vi "p1.vi"() -> ()   [LabVIEW 2021, in "d14.lvlib"]
uses:
  d14.lvlib
  AOC/AOC.lvlib
panel:
  out "XY Graph":cluster{"Left out":u32[], "Top out":u32[]}[](graph)
  out "Answer":i32
  in  "Example":string="498,4 -> 498,6 -> 496,6\n503,4 -> 502,4 -> 502,9 -> 494,9"
  in  "Example":bool
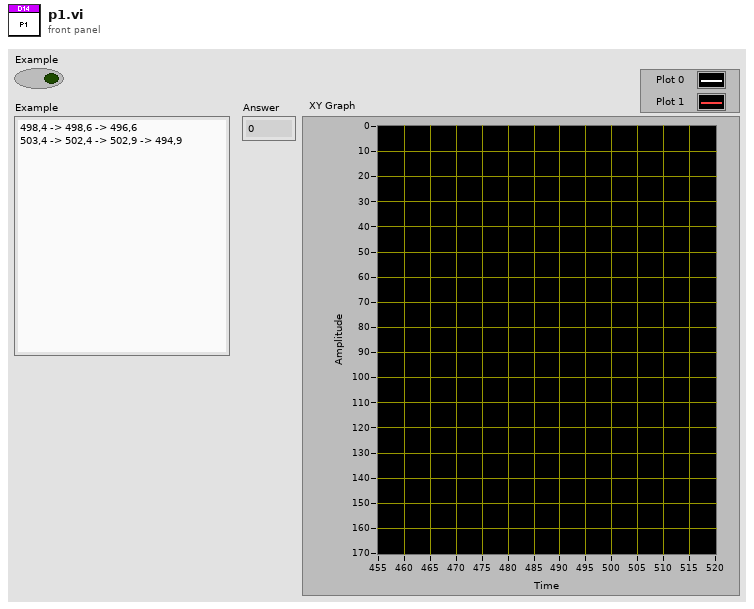
[diagram p1: front panel]
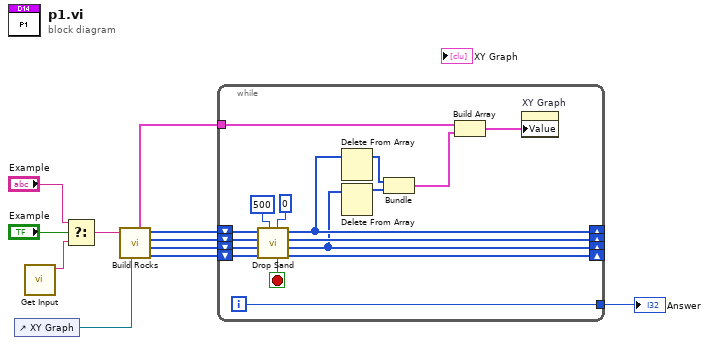
[diagram p0: block diagram]
diagram:
  n1 = control-ref of="XY Graph"() -> (w1:refnum<vi>)
  n2 = call "Get Input.vi"() -> ("Input"=w11:string)  [unwired: 11 in]
  n3 = Select(t="Example", s="Example", f=w11) -> (s? t:f=w10:string)
  n4 = call "Build Rocks.vi"("reference"=w1, "Input"=w10) -> ("Bottom"=w3:i32[], "Top"=w5:i32[], "Right"=w4:i32[], "Left"=w6:i32[], "Rocks"=w2:cluster{u32[], u32[]})  [unwired: 4 in, 1 out]
  n5 = while {
    tunnel: [w23] -> w7
    shift-right: [w18] -> _
    shift-left: w6 -> [w27]
    shift-right: [w20] -> _
    shift-left: w4 -> [w26]
    shift-right: [w17] -> _
    shift-left: w5 -> [w28]
    shift-right: [w19] -> _
    shift-left: w3 -> [w25]
    tunnel: w2 -> [w14]
    i -> [w23]
    stop <- w24 stop-if-true
    n6 = call "Drop Sand.vi"("Y in"=0, "X in"=500, "Bottom in"=w25, "Top in"=w28, "Right in"=w26, "Left in"=w27) -> ("Bottom out"=w19:i32[], "Top out"=w17:i32[], "Right out"=w20:i32[], "Left out"=w18:i32[], "falling forever?"=w24:bool)  [unwired: 1 in]
    n7 = Delete From Array(array=w18) -> (array with subset deleted=w16:i32[])  [unwired: 2 in, 1 out]
    n8 = Delete From Array(array=w17) -> (array with subset deleted=w15:i32[])  [unwired: 2 in, 1 out]
    n9 = Bundle("Left out"=w16, "Top out"=w15) -> (w13:cluster{"Left out":i32[], "Top out":i32[]})  [unwired: 1 in]
    n10 = Build Array(w14, w13) -> (w12:cluster{"Left out":u32[], "Top out":u32[]}[])
    n11 = property on="XY Graph" class="XYGraph (strict)"("Value"=w12) -> ()  [unwired: 2 in, 2 out]
  }
  "Answer" <- w7
